vi "makeOverlayText.vi"(10 "ADAMspecs":T1(array[cluster])) -> (2 "OverlayText":string)   [LabVIEW 2021]
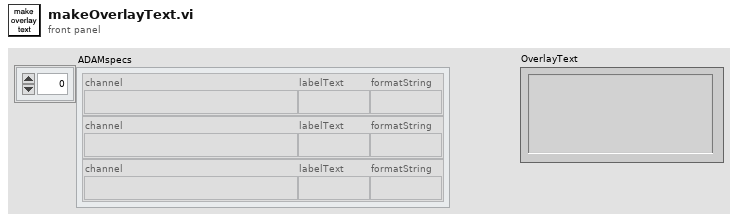
[diagram p1: front panel]
types:
  T1 = cluster{"channel":string, "labelText":string, "formatString":string}[]
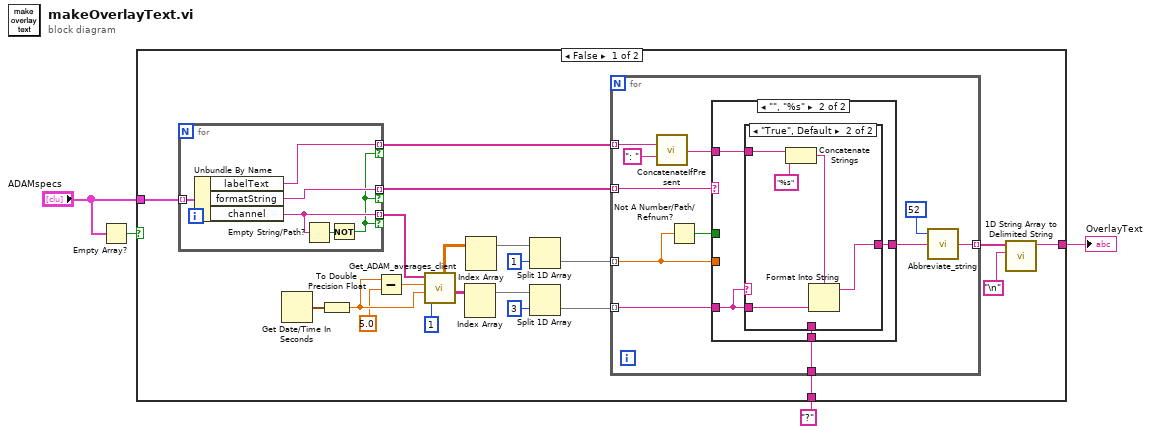
[diagram p0: block diagram]
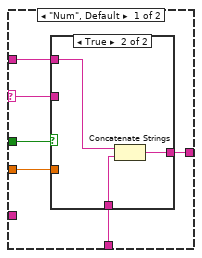
[diagram p2: hidden frame]
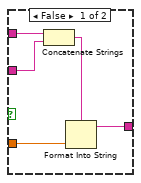
[diagram p3: hidden frame]
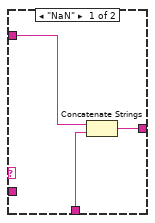
[diagram p4: hidden frame]
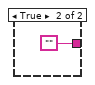
[diagram p5: hidden frame]
diagram:
  n1 = Empty Array?(array="ADAMspecs") -> (empty?=w3:bool)
  n2 = case shown="False" w3 {
    tunnel: "ADAMspecs" -> [w25 _]
    tunnel: [w14 ""] -> w4
    tunnel: "?" ("string") -> [w5 _]
    frame False {
      n3 = for {
        tunnel: w25 -> [w68] mode=indexing
        tunnel: [w66] -> w22 mode=indexing if=w63
        tunnel: [w65] -> w8 mode=indexing if=w63
        tunnel: [w64] -> w7 mode=indexing if=w63
        n4 = Unbundle By Name(w68) -> ("labelText"=w64:string, "formatString"=w65:string, "channel"=w66:string)
        n5 = Empty String/Path?(string/path=w66) -> (empty?=w67:bool)
        n6 = Not(x=w67) -> (.not. x?=w63:bool)
      }
      n7 = Get Date/Time In Seconds() -> (seconds since 1Jan1904=w18:timestamp)
      n8 = To Double Precision Float(number=w18) -> (double precision float=w21:dbl)
      n9 = Subtract(x=w21, y=5.0) -> (x-y=w20:dbl)
      n10 = call "Get_ADAM_averages_client.vi"("No of averages"=1, "End time"=w21, "Start time"=w20, "ADAM Ch Names"=w22) -> ("Values"=w16:string[][], "DBL values"=w11:dbl[][])  [unwired: 3 in, 3 out]
      n11 = Index Array(array=w16) -> (element=w23:string[])  [unwired: 2 in]
      n12 = Index Array(array=w11) -> (element=w13:dbl[])  [unwired: 2 in]
      n13 = Split 1D Array(array=w13, index=1) -> (second subarray=w10:dbl[])  [unwired: 1 out]
      n14 = Split 1D Array(array=w23, index=3) -> (second subarray=w9:string[])  [unwired: 1 out]
      n15 = for {
        tunnel: w10 -> [w31] mode=indexing
        tunnel: w9 -> [w35] mode=indexing
        tunnel: w8 -> [w36] mode=indexing
        tunnel: w7 -> [w34] mode=indexing
        tunnel: [w27] -> w6 mode=indexing
        tunnel: w5 -> [w29]
        n16 = call "ConcatenateIfPresent.vi"("prependString"=w34, "appendString"=": " ("string")) -> ("outputString"=w32:string)  [unwired: 13 in]
        n17 = Not A Number/Path/Refnum?(number/path/refnum=w31) -> (NaN/Path/Refnum?=w30:bool)
        n18 = case shown="\"\", \"%s\"" w36 {
          selector: w36 -> [w40 _]
          tunnel: w35 -> [_ w52]
          tunnel: w32 -> [w42 w54]
          tunnel: w31 -> [w41 _]
          tunnel: [w39 w53] -> w28
          tunnel: w30 -> [w38 _]
          tunnel: w29 -> [w37 w51]
          frame "Num", Default {
            n19 = case shown="True" w38 {
              tunnel: w42 -> [w47 w50]
              tunnel: w41 -> [w45 _]
              tunnel: w40 -> [w44 _]
              tunnel: [w43 w49] -> w39
              tunnel: w37 -> [_ w48]
              frame False {
                n20 = Concatenate Strings(w47, w44) -> (w46:string)
                n21 = Format Into String(format string=w46, w45) -> (resulting string=w43:string)  [unwired: 2 in, 1 out]
              }
              frame True {
                n22 = Concatenate Strings(w50, w48) -> (w49:string)
              }
            }
          }
          frame "", "%s" {
            n23 = case shown="\"True\", Default" w52 {
              tunnel: w52 -> [_ w62]
              tunnel: w54 -> [w57 w61]
              tunnel: [w56 w58] -> w53
              tunnel: w51 -> [w55 _]
              frame "NaN" {
                n24 = Concatenate Strings(w57, w55) -> (w56:string)
              }
              frame "True", Default {
                n25 = Concatenate Strings(w61, "%s" ("string")) -> (w59:string)
                n26 = Format Into String(format string=w59, w62) -> (resulting string=w58:string)  [unwired: 2 in, 1 out]
              }
            }
          }
        }
        n27 = call "Abbreviate_string.vi"("Input String"=w28, "Max String Length"=52) -> ("Output String"=w27:string)  [unwired: 1 in, 2 out]
      }
      n28 = call <vilib>:"1D String Array to Delimited String.vi"("delimiter"="\n", "string array"=w6) -> ("delimited string"=w14:string)  [unwired: 9 in]
    }
    frame True {
    }
  }
  "OverlayText" <- w4
